vi "Read Temperature (F).vi"(8 "error in (no error)":errorcluster, 11 "LPS Barometric Pressure Sensor in":refnum<class "LPS Barometric Pressure Sensor.lvclass">) -> (0 "error out":errorcluster, 2 "Temperature (F)":dbl, 3 "LPS Barometric Pressure Sensor out":refnum<class "LPS Barometric Pressure Sensor.lvclass">)   [LabVIEW 2020, in "LPS Barometric Pressure Sensor.lvclass"]
uses:
  LPS Barometric Pressure Sensor.lvclass
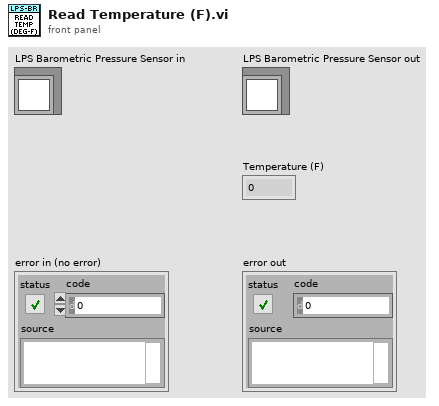
[diagram p1: front panel]
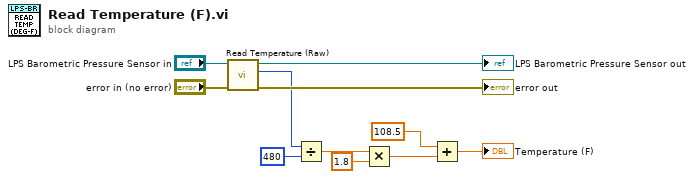
[diagram p0: block diagram]
diagram:
  n1 = call-dynamic "Read Temperature (Raw).vi"("error in (no error)"="error in (no error)", "LPS Barometer in"="LPS Barometric Pressure Sensor in") -> ("error out"=→"error out":errorcluster, "Raw Temperature"=w7:i16, "LPS Barometer out"=→"LPS Barometric Pressure Sensor out":refnum<class "LPS Barometric Pressure Sensor.lvclass">)  [unwired: 7 in]
  n2 = Divide(x=w7, y=i16 480) -> (x/y=w5:dbl)
  n3 = Multiply(x=w5, y=1.8) -> (x*y=w2:dbl)
  n4 = Add(x=108.5, y=w2) -> (x+y=→"Temperature (F)":dbl)
